vi "Swerve Wheel.vi"(7 "Wheel":T1(ring), 10 "Inputs":dbl[](array[numeric])) -> (1 "Speed":dbl, 2 "Motor Output":dbl)   [LabVIEW 2016]
uses:
  <vilib>/Rock Robotics/Network Tables/NT Read Number.vi
  <vilib>/Rock Robotics/Network Tables/NT Write Number.vi
  <vilib>/addons/control/pid/pid.llb/PID (DBL).vi
  <vilib>/addons/control/pid/NI_PID_pid.lvlib
panel:
  out "PID Values":cluster{"P":dbl, "I":dbl, "D":dbl}
  # "Swerve Wheel Control\nFRC Team 34"
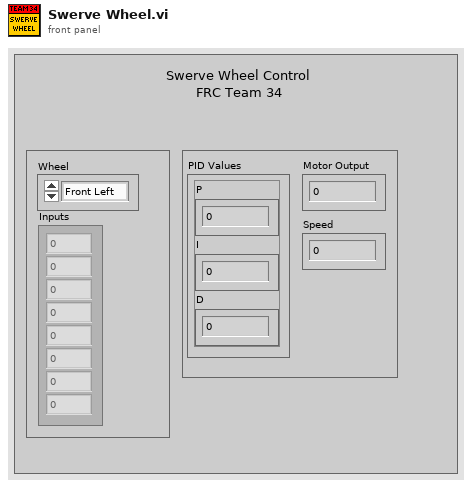
[diagram p1: front panel]
types:
  T1 = enum16{"Front Left", "Front Right", "Back Left", "Back Right"}
  T2 = enum16{"Z", "Y", "X", "Rot. Point X", "Rot. Point Y", "Width/2", "Max", "Length/2"}
  T3 = enum16{"Z Axis", "Y", "X", "Rot. Point X", "Rot. Point Y", "Width/2", "Max", "Length/2"}
  T4 = typedef "WPI_MotorControlDeviceRef.ctl" = cluster{"DeviceStatus":errorcluster, "Type":T5, "PWM":cluster{"PWM Channel":T6, "DeadBand":T7}, "CAN":cluster{"Device Number":u8, "SetOutput VI Ref":variant, "GetOutput VI Ref":variant, "Enable VI Ref":variant, "Disable VI Ref":variant, "Data":variant}, "Invert":bool}
  T5 = typedef "WPI_MotorControlType.ctl" = enum16{"PWM", "CAN"}
  T6 = typedef "FPGA_DIOPWMChannel.ctl" = enum8{"PWM 0", "PWM 1", "PWM 2", "PWM 3", "PWM 4", "PWM 5", "PWM 6", "PWM 7", "PWM 8", "PWM 9", "PWM MXP 0", "PWM MXP 1", "PWM MXP 2", "PWM MXP 3", "PWM MXP 4", "PWM MXP 5", "PWM MXP 6", "PWM MXP 7", "PWM MXP 8", "PWM MXP 9", "Invalid"}
  T7 = typedef "WPI_PWMDeadband.ctl" = cluster{"Name":string, "maxPositivePwm":i32, "minPositivePwm":i32, "centerPwm":i32, "maxNegativePwm":i32, "minNegativePwm":i32, "angularRange":u16}
  T8 = typedef "WPI_EncoderDevRef.ctl" = cluster{"DevStatus":errorcluster, "EncoderIndex":T9, "CounterIndex":T10, "DistancePerCount":dbl, "Decoding Type":T11}
  T9 = typedef "FPGA_EncoderIdx.ctl" = enum8{"Enc 0", "Enc 1", "Enc 2", "Enc 3", "Enc 4", "Enc 5", "Enc 6", "Enc 7", "Invalid"}
  T10 = typedef "FPGA_CounterCtrSystemIndex.ctl" = enum8{"Ctr 0", "Ctr 1", "Ctr 2", "Ctr 3", "Ctr 4", "Ctr 5", "Ctr 6", "Ctr 7", "Invalid"}
  T11 = typedef "WPI_EncoderType.ctl" = enum16{"1x", "2x", "4x"}
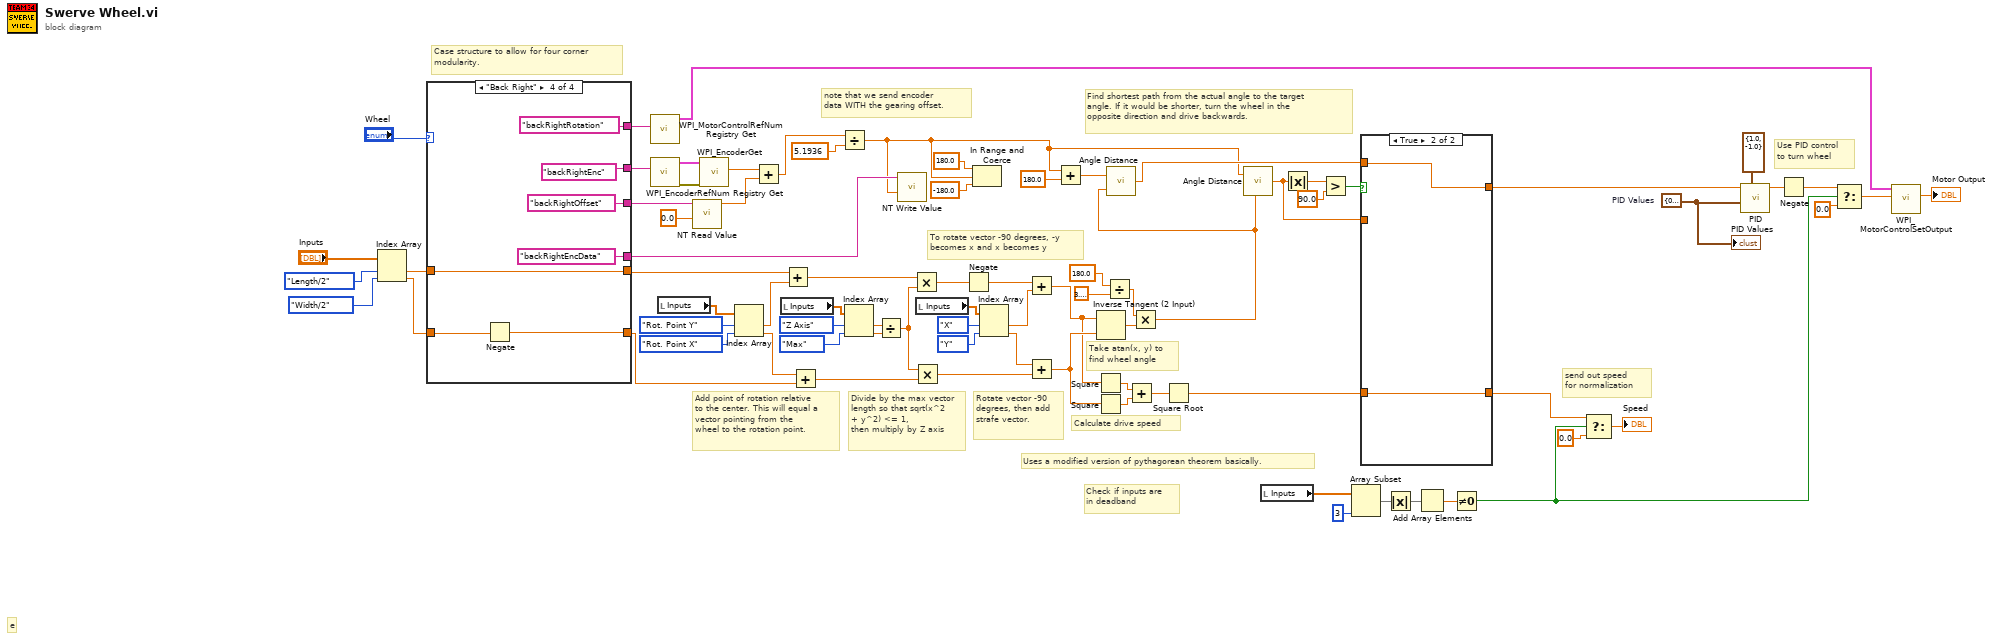
[diagram p0: block diagram]
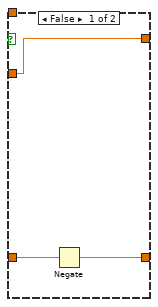
[diagram p2: hidden frame]
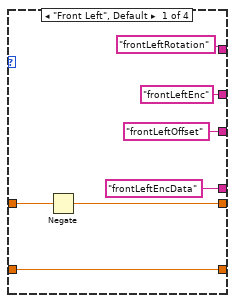
[diagram p3: hidden frame]
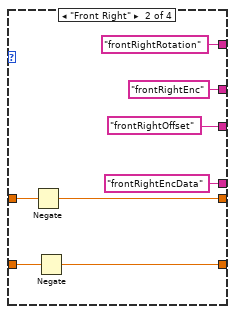
[diagram p4: hidden frame]
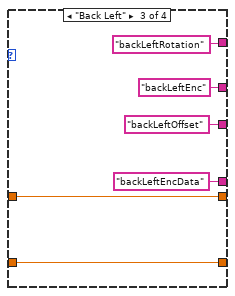
[diagram p5: hidden frame]
diagram:
  w1 = cluster{"P":dbl, "I":dbl, "D":dbl} {"P"=0.1, "I"=0.0, "D"=0.0}  # PID Values
  # "Uses a modified version of pythagorean theorem basically."
  # "e"
  # "note that we send encoder \ndata WITH the gearing offset."
  # "Case structure to allow for four corner\nmodularity."
  # "To rotate vector -90 degrees, -y becomes x and x becomes y"
  # "send out speed\nfor normalization"
  # "Use PID control\nto turn wheel"
  # "Find shortest path from the actual angle to the target angle. If it would be shorter, turn the wheel in the opposite direction and drive backwards."
  # "Divide by the max vector length so that sqrt(x^2 + y^2) <= 1,\nthen multiply by Z axis"
  # "Add point of rotation relative to the center. This will equal a vector pointing from the\nwheel to the rotation point."
  # "Check if inputs are\nin deadband"
  # "Take atan(x, y) to find wheel angle"
  # "Calculate drive speed"
  # "Rotate vector -90 degrees, then add strafe vector."
  n1 = Index Array(array="Inputs", index #1=T2."Length/2", index #2=T2."Width/2") -> (element #1=w75:dbl, element #2=w74:dbl)
  n2 = case shown="\"Back Right\"" "Wheel" {
    tunnel: w75 -> [w86 w94 w100 w107]
    tunnel: w74 -> [w84 w92 w99 w106]
    tunnel: [w85 w93 w100 w107] -> w42
    tunnel: [w84 w91 w99 w105] -> w41
    tunnel: ["frontLeftRotation" "frontRightRotation" "backLeftRotation" "backRightRotation"] -> w73
    tunnel: ["frontLeftEnc" ("refnum name") "frontRightEnc" ("refnum name") "backLeftEnc" ("refnum name") "backRightEnc" ("refnum name")] -> w54
    tunnel: ["frontLeftOffset" ("Name") "frontRightOffset" ("Name") "backLeftOffset" ("Name") "backRightOffset" ("Name")] -> w50
    tunnel: ["frontLeftEncData" ("Name") "frontRightEncData" ("Name") "backLeftEncData" ("Name") "backRightEncData" ("Name")] -> w10
    frame "Front Left", Default {
      n3 = Negate(x=w86) -> (-x=w85:dbl)
    }
    frame "Front Right" {
      n4 = Negate(x=w94) -> (-x=w93:dbl)
      n5 = Negate(x=w92) -> (-x=w91:dbl)
    }
    frame "Back Left" {
    }
    frame "Back Right" {
      n6 = Negate(x=w106) -> (-x=w105:dbl)
    }
  }
  n7 = call <vilib>:"WPI_MotorControlRefNum Registry Get.vi"("refnum name"=w73) -> ("MotorControlDevRef"=w17:T4)  [unwired: 9 in, 1 out]
  n8 = call <vilib>:"WPI_EncoderRefNum Registry Get.vi"("refnum name"=w54) -> ("error out"=w53:errorcluster, "EncoderDevRef"=w52:T8)  [unwired: 9 in]
  n9 = local read "Inputs"() -> (w47:dbl[])
  n10 = call-poly <vilib>:"NT Read Value.vi"("Default Value"=0.0, "Name"=w50) -> ("Numeric"=w45:dbl)  [unwired: 8 in, 1 out]
  n11 = call <vilib>:"WPI_EncoderGet.vi"("error in (no error)"=w53, "EncoderDevRef"=w52) -> ("Distance"=w46:dbl)  [unwired: 4 in, 5 out]
  n12 = Index Array(array=w47, index #1=T2."Rot. Point Y", index #2=T2."Rot. Point X") -> (element #1=w43:dbl, element #2=w44:dbl)
  n13 = Add(x=w46, y=w45) -> (x+y=w8:dbl)
  n14 = local read "Inputs"() -> (w55:dbl[])
  n15 = Add(x=w42, y=w43) -> (x+y=w40:dbl)
  n16 = Add(x=w44, y=w41) -> (x+y=w65:dbl)
  n17 = Divide(x=w8, y=5.1936) -> (x/y=w5:dbl)
  n18 = Index Array(array=w55, index #1=T3."Z Axis", index #2=T2."Max") -> (element #1=w12:dbl, element #2=w11:dbl)
  n19 = Divide(x=w12, y=w11) -> (x/y=w64:dbl)
  n20 = call-poly <vilib>:"NT Write Value.vi"("Numeric"=w5, "Name"=w10) -> ()  [unwired: 9 in, 1 out]
  n21 = Multiply(x=w40, y=w64) -> (x*y=w57:dbl)
  n22 = Multiply(x=w64, y=w65) -> (x*y=w60:dbl)
  n23 = local read "Inputs"() -> (w15:dbl[])
  n24 = Negate(x=w57) -> (-x=w56:dbl)
  n25 = In Range and Coerce(upper limit=180.0, x=w5, lower limit=-180.0 ("upper limit")) -> ()  [unwired: 2 out]
  n26 = Index Array(array=w15, index #1=T2."X", index #2=T2."Y") -> (element #1=w14:dbl, element #2=w13:dbl)
  n27 = Add(x=w56, y=w14) -> (x+y=w58:dbl)
  n28 = Add(x=w13, y=w60) -> (x+y=w59:dbl)
  n29 = Add(x=w5, y=180.0) -> (x+y=w37:dbl)
  n30 = Inverse Tangent (2 Input)(1:w59, 2:w58) -> (0:w72:dbl)
  n31 = Square(x=w58) -> (x^2=w61:dbl)
  n32 = Square(x=w59) -> (x^2=w71:dbl)
  n33 = Divide(x=180.0 ("y"), y=3.141592653589793) -> (x/y=w69:dbl)
  n34 = Add(x=w61, y=w71) -> (x+y=w70:dbl)
  n35 = Multiply(x=w69, y=w72) -> (x*y=w38:dbl)
  n36 = call "Angle Distance.vi"("Target Angle"=w38, "Current Angle"=w37) -> ("Distance"=w30:dbl)
  n37 = Square Root(x=w70) -> (sqrt(x)=w32:dbl)
  n38 = call "Angle Distance.vi"("Target Angle"=w38, "Current Angle"=w5) -> ("Distance"=w31:dbl)
  n39 = local read "Inputs"() -> (w26:dbl[])
  n40 = Absolute Value(x=w31) -> (abs(x)=w35:dbl)
  n41 = Greater?(x=w35, y=90.0) -> (0:w33:bool)
  n42 = Array Subset(array=w26, length=3) -> (w28:dbl[])  [unwired: 1 in]
  n43 = case shown="True" w33 {
    tunnel: w32 -> [w109 w111]
    tunnel: w31 -> [w110 _]
    tunnel: w30 -> [_ w112]
    tunnel: [w108 w111] -> w24
    tunnel: [w110 w112] -> w2
    frame False {
      n44 = Negate(x=w109) -> (-x=w108:dbl)
    }
    frame True {
    }
  }
  n45 = Absolute Value(x=w28) -> (abs(x)=w27:dbl[])
  n46 = Add Array Elements(numeric array=w27) -> (sum=w29:dbl)
  n47 = Not Equal To 0?(x=w29) -> (x != 0?=w16:bool)
  n48 = Select(t=w24, s=w16, f=0.0) -> (s? t:f=→"Speed":dbl)
  n49 = call-poly <vilib>:"PID.vi"("output range"=cluster{"output high":dbl, "output low":dbl} {"output high"=1.0, "output low"=-1.0}, "PID gains"=w1, "setpoint"=w2) -> ("output"=w20:dbl)  [unwired: 7 in, 1 out]
  n50 = Negate(x=w20) -> (-x=w18:dbl)
  n51 = Select(t=w18, s=w16, f=0.0) -> (s? t:f=w6:dbl)
  n52 = call <vilib>:"WPI_MotorControlSetOutput.vi"("Output"=w6, "MotorControlDevRef"=w17) -> ("Motor Output"=→"Motor Output":dbl)  [unwired: 7 in, 2 out]
  "PID Values" <- w1
